vi "CRYView Pic Convert to VariantList.vi"(7 "sAction":string, 10 "pRefListTF":refnum<vi>[](array[refnum]), 11 "pRefListVI":refnum<vi>[](array[refnum])) -> (3 "RefList_Out":variant[](array[variant]))   [LabVIEW 2013]
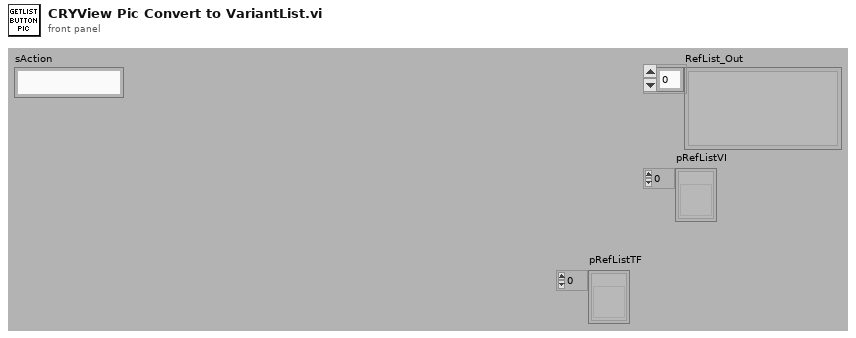
[diagram p1: front panel]
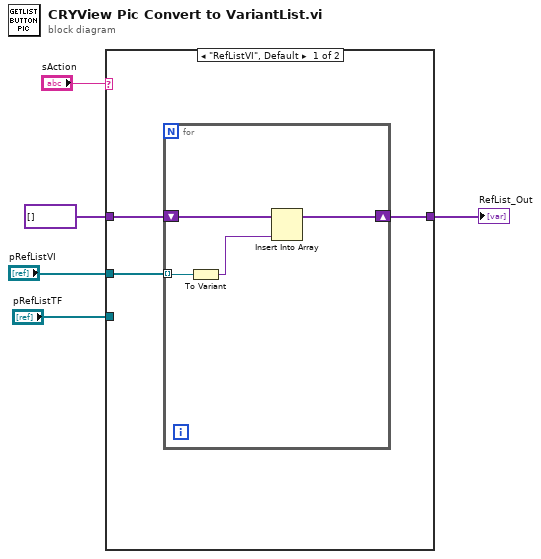
[diagram p0: block diagram]
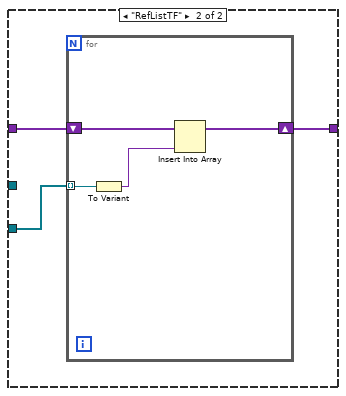
[diagram p2: hidden frame]
diagram:
  n1 = case shown="\"RefListVI\", Default" "sAction" {
    tunnel: variant[] [] -> [w8 w15]
    tunnel: [w7 w14] -> w4
    tunnel: "pRefListVI" -> [w6 _]
    tunnel: "pRefListTF" -> [_ w13]
    frame "RefListVI", Default {
      n2 = for {
        shift-right: [w10] -> w7
        shift-left: w8 -> [w11]
        tunnel: w6 -> [w12] mode=indexing
        n3 = To Variant(anything=w12) -> (Variant=w9:variant)
        n4 = Insert Into Array(array=w11, new element=w9) -> (w10:variant[])  [unwired: 1 in]
      }
    }
    frame "RefListTF" {
      n5 = for {
        shift-right: [w17] -> w14
        shift-left: w15 -> [w18]
        tunnel: w13 -> [w19] mode=indexing
        n6 = To Variant(anything=w19) -> (Variant=w16:variant)
        n7 = Insert Into Array(array=w18, new element=w16) -> (w17:variant[])  [unwired: 1 in]
      }
    }
  }
  "RefList_Out" <- w4
